vi "write_command.vi"(8 "error in (no error)":errorcluster, 9 "read (T)":bool=TRUE, 10 "string to write":string, 11 "LightSourceMH110125Tsunami in":refnum<class "LightSourceMH110125Tsunami.lvclass">) -> (0 "error out":errorcluster, 2 "read string":string, 3 "LightSourceMH110125Tsunami out":refnum<class "LightSourceMH110125Tsunami.lvclass">)   [LabVIEW 2010, in "LightSourceMH110125Tsunami.lvclass"]
uses:
  LightSourceMH110125Tsunami.lvclass
  LightSourceMH110125Tsunami.lvclass/LightSourceMH110125Tsunami.ctl
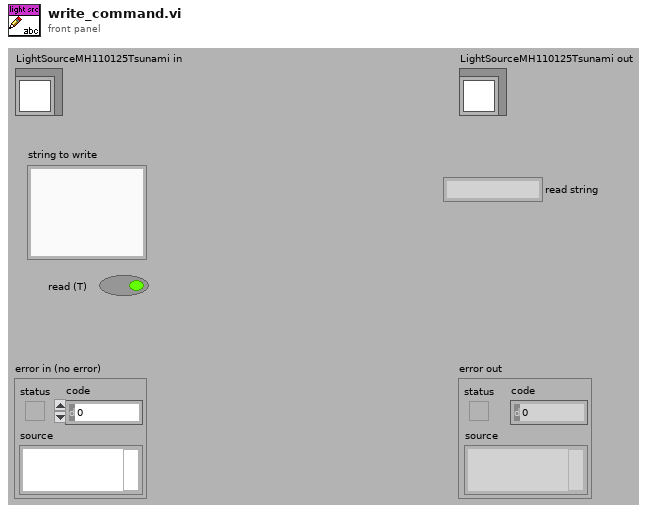
[diagram p1: front panel]
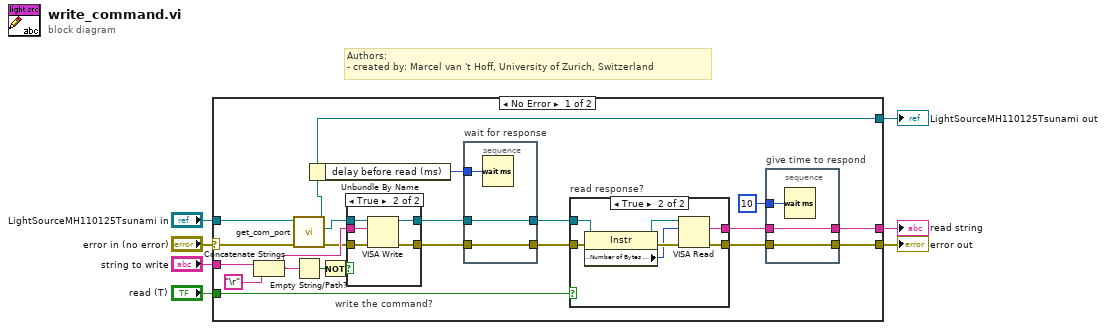
[diagram p0: block diagram]
diagram:
  # "Authors: \n- created by: Marcel van 't Hoff, University of Zurich, Switzerland"
  n1 = case shown="No Error" "error in (no error)" {
    selector: "error in (no error)" -> [w27 w51]
    tunnel: [w9 w51] -> w6
    tunnel: [w19 w50] -> w4
    tunnel: "LightSourceMH110125Tsunami in" -> [w28 w50]
    tunnel: "string to write" -> [w24 _]
    tunnel: "read (T)" -> [w13 _]
    tunnel: [w8 _] -> w1
    frame No Error {
      n2 = Concatenate Strings(w24, "\r") -> (w22:string)
      n3 = call-dynamic "get_com_port.vi"("error in (no error)"=w27, "LightSourceMH110125Tsunami in"=w28) -> ("error out"=w20:errorcluster, "comm port"=w23:refnum<visa-resource-name>, "LightSourceMH110125Tsunami out"=w19:refnum<class "LightSourceMH110125Tsunami.lvclass">)  [unwired: 7 in]
      n4 = Empty String/Path?(string/path=w22) -> (empty?=w25:bool)
      n5 = Unbundle By Name(w19) -> ("delay before read (ms)"=w16:u32)
      n6 = Not(x=w25) -> (.not. x?=w21:bool)
      n7 = case "write the command?" shown="True" w21 {
        tunnel: [w44 w49] -> w17
        tunnel: w23 -> [w43 w48]
        tunnel: w20 -> [w44 w47]
        tunnel: [w43 w46] -> w18
        tunnel: w22 -> [_ w45]
        frame False {
        }
        frame True {
          n8 = VISA Write(VISA resource name=w48, write buffer=w45, error in (no error)=w47) -> (VISA resource name out=w46:refnum<visa-resource-name>, error out=w49:errorcluster)  [unwired: 1 out]
        }
      }
      n9 = stacked-sequence "wait for response" {
        tunnel: w17 -> [w42]
        tunnel: [w42] -> w15
        tunnel: w18 -> [w41]
        tunnel: [w41] -> w14
        tunnel: w16 -> [w40]
        frame #0 {
          n10 = Wait (ms)(milliseconds to wait=w40) -> ()  [unwired: 1 out]
        }
      }
      n11 = case "read response?" shown="True" w13 {
        tunnel: w15 -> [w32 w36]
        tunnel: [w32 w39] -> w12
        tunnel: w14 -> [_ w38]
        tunnel: [_ w33] -> w11
        frame False {
        }
        frame True {
          n12 = property class="Instr"(reference=w38, error in=w36) -> (reference out=w37:refnum<visa-resource-name>, error out=w35:errorcluster, "Serial Settings:Number of Bytes at Serial Port"=w34:u32)
          n13 = VISA Read(VISA resource name=w37, byte count=w34, error in (no error)=w35) -> (read buffer=w33:string, error out=w39:errorcluster)  [unwired: 2 out]
        }
      }
      n14 = stacked-sequence "give time to respond" {
        tunnel: w12 -> [w31]
        tunnel: [w31] -> w9
        tunnel: w11 -> [w30]
        tunnel: [w30] -> w8
        tunnel: u32 10 ("delay before read (ms)") -> [w29]
        frame #0 {
          n15 = Wait (ms)(milliseconds to wait=w29) -> ()  [unwired: 1 out]
        }
      }
    }
    frame Error {
    }
  }
  "error out" <- w6
  "LightSourceMH110125Tsunami out" <- w4
  "read string" <- w1
